vi "GetCurrentTarget.vi"(0 "object in":refnum<class "Navigation.lvclass">, 2 "Dest_array":T1(array[cluster]), 4 "maxAngle":dbl format="%#_13g", 5 "error in (no error)":errorcluster) -> (14 "object out":refnum<class "Navigation.lvclass">, 17 "Target":dbl[](array[numeric]), 19 "error out":errorcluster)   [LabVIEW 2023, in "Navigation.lvclass"]
uses:
  Navigation.lvclass
  Utilities_class/Utilities.lvclass
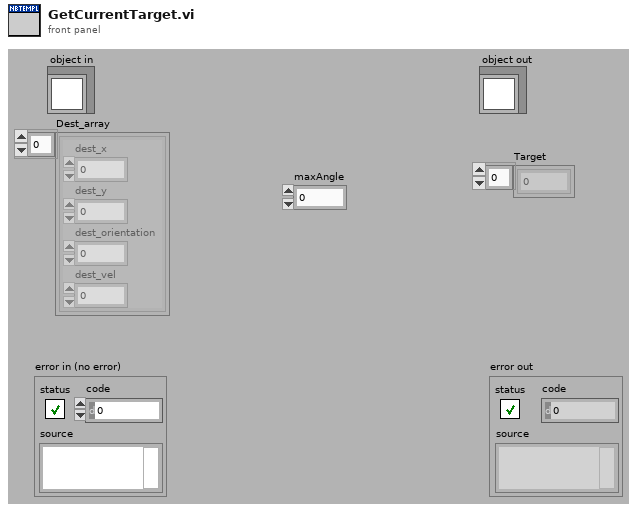
[diagram p1: front panel]
types:
  T1 = cluster{"dest_x":dbl, "dest_y":dbl, "dest_orientation":dbl, "dest_vel":dbl}[]
  T2 = cluster{"dest_x":dbl, "dest_y":dbl, "dest_orientation":dbl, "dest_vel":dbl}
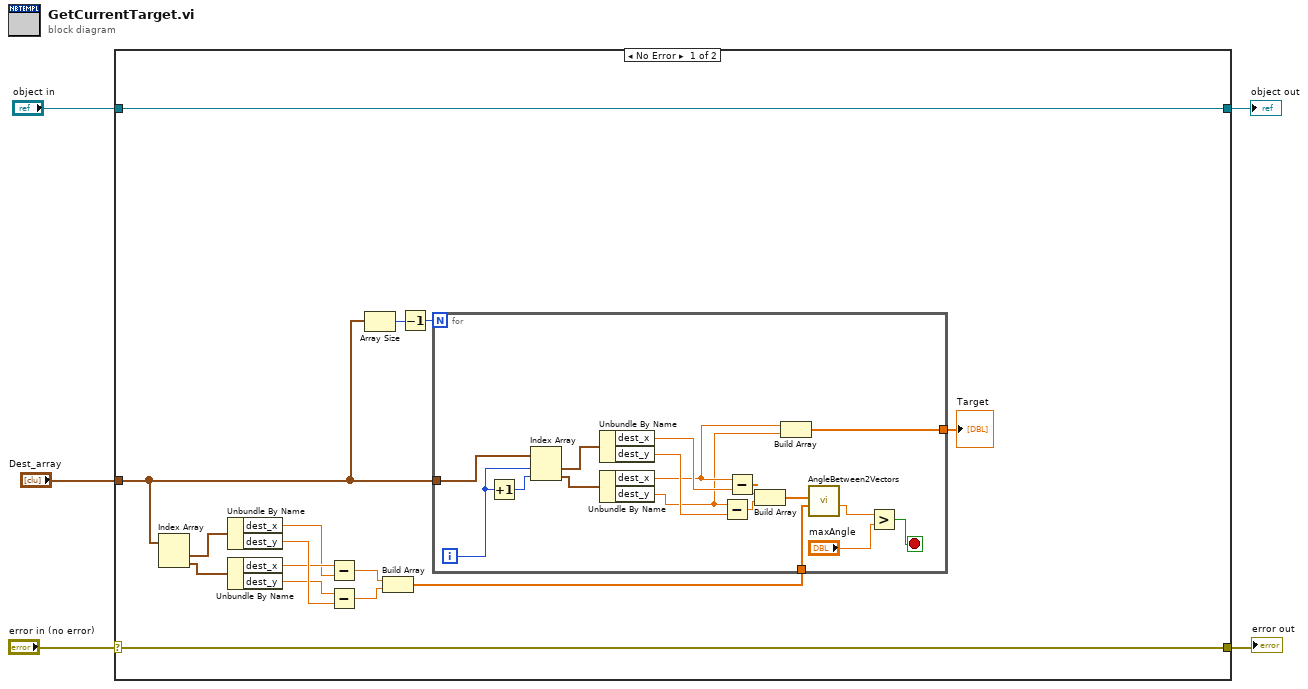
[diagram p0: block diagram]
diagram:
  n1 = case shown="No Error" "error in (no error)" {
    selector: "error in (no error)" -> [w19 w39]
    tunnel: [w19 w39] -> w4
    tunnel: [w20 w38] -> w2
    tunnel: "object in" -> [w20 w38]
    tunnel: "Dest_array" -> [w9 _]
    frame No Error {
      n2 = Index Array(array=w9) -> (element #1=w10:T2, element #2=w11:T2)  [unwired: 2 in]
      n3 = Unbundle By Name(w10) -> ("dest_x"=w8:dbl, "dest_y"=w14:dbl)
      n4 = Unbundle By Name(w11) -> ("dest_x"=w12:dbl, "dest_y"=w13:dbl)
      n5 = Subtract(x=w12, y=w8) -> (x-y=w15:dbl)
      n6 = Subtract(x=w13, y=w14) -> (x-y=w16:dbl)
      n7 = Array Size(array=w9) -> (size(s)=w18:i32)
      n8 = Build Array(w15, w16) -> (w7:dbl[])
      n9 = Decrement(x=w18) -> (x-1=w17:i32)
      n10 = for {
        N: w17 -> [_]
        tunnel: w9 -> [w37]
        tunnel: w7 -> [w29]
        tunnel: [w23] -> w6
        i -> [w36]
        stop <- w26 stop-if-true
        n11 = Increment(x=w36) -> (x+1=w35:i32)
        n12 = Index Array(array=w37, index #1=w36, index #2=w35) -> (element #1=w34:T2, element #2=w33:T2)
        n13 = Unbundle By Name(w34) -> ("dest_x"=w32:dbl, "dest_y"=w31:dbl)
        n14 = Unbundle By Name(w33) -> ("dest_x"=w22:dbl, "dest_y"=w21:dbl)
        n15 = Subtract(x=w21, y=w31) -> (x-y=w24:dbl)
        n16 = Subtract(x=w22, y=w32) -> (x-y=w25:dbl)
        n17 = Build Array(w25, w24) -> (w30:dbl[])
        n18 = Build Array(w22, w21) -> (w23:dbl[])
        n19 = call "AngleBetween2Vectors.vi"("Array 1"=w29, "Array 2"=w30) -> ("angleInDegrees"=w28:dbl)  [unwired: 6 in, 3 out]
        n20 = Greater?(x=w28, y="maxAngle") -> (0:w26:bool)
      }
      "Target" <- w6
    }
    frame Error {
    }
  }
  "error out" <- w4
  "object out" <- w2
